vi "Instrument_Setting.vi"(8 "错误输入（无错误）":errorcluster, 9 "id":string[](array[string]), 10 "Get_USB_Resouce":string[](array[string]), 11 "Address Cluster":T2={"SPU"=refnum, "MPM"=[], "Port_Count"=0.0, "MPM_Count"=0.0, "SPU_Resource"=[], "USB_Resource"=[], "MPM_Communicater"="", "MPM_Count"=0.0, "MPM_Address"=[], "MPM_Portnumber"=[], "SPU_DeviveID"="", "MPM_communcation_method"=[], "TSL_sweepstartwave"=0.0, "TSL_sweepstopwave"=0.0, "TSL_Address"="", "TSL_Communicater"="", "TSL"=refnum, "tsl_communcation_method"=3, "TSL_Portnumber"=0.0, "PCU"=refnum, "PCU_Communicater"="", "PCU_Address"="", "PCU_Portnumber"=0.0, "PCU_useing_internal_DAQ"=FALSE, "PCU_communcation_method"=0} {"PCU_communcation_method" items=["GPIB", "C232C", "TCPIP", "USB"]; "tsl_communcation_method" items=["GPIB", "C232C", "TCPIP", "USB"]; "MPM_communcation_method" items=["GPIB", "C232C", "TCPIP", "USB"]}) -> (0 "错误输出":errorcluster, 3 "Address Cluster out":T2={"SPU"=refnum, "MPM"=[], "Port_Count"=0.0, "MPM_Count"=0.0, "SPU_Resource"=[], "USB_Resource"=[], "MPM_Communicater"="", "MPM_Count"=0.0, "MPM_Address"=[], "MPM_Portnumber"=[], "SPU_DeviveID"="", "MPM_communcation_method"=[], "TSL_sweepstartwave"=0.0, "TSL_sweepstopwave"=0.0, "TSL_Address"="", "TSL_Communicater"="", "TSL"=refnum, "tsl_communcation_method"=3, "TSL_Portnumber"=0.0, "PCU"=refnum, "PCU_Communicater"="", "PCU_Address"="", "PCU_Portnumber"=0.0, "PCU_useing_internal_DAQ"=FALSE, "PCU_communcation_method"=0} {"PCU_communcation_method" items=["GPIB", "C232C", "TCPIP", "USB"]; "tsl_communcation_method" items=["GPIB", "C232C", "TCPIP", "USB"]; "MPM_communcation_method" items=["GPIB", "C232C", "TCPIP", "USB"]})   [LabVIEW 2017]
doc: "Setting Form"
uses:
  CTL/Address Cluster.ctl
  D:/test/PDLSTS/LV_PDL_Sample/DLL/InstrumentDLL.dll
  DLL/InstrumentDLL.dll
panel:
  in  "txtpcu_ipadd":string caption="IP Address"
  in  "txtpcu_lanport":i32 caption="LAN Port"
  in  "txtpcu_gpibadd":i32=1 caption="GPIB Address"
  in  "cmbpcu_usbresource":u16(ring) caption="Usb resouce"
  in  "Communication_PCU":T1(radio) caption="Communication"
  in  "Product_PCU":enum32{"rdopcu100", "rdopcu110"}(radio) caption="Product"
  out "Boolean":bool=TRUE
  in  "Port_Count":i32
  in  "btnconnect":bool
  in  "cmbSPU_dev":u16(ring) caption="SPU" items=["Dev8"]
  in  "IP Address_MPM 2":string caption="IP Address"
  in  "LAN Port_MPM 2":dbl caption="LAN Port"
  in  "GPIB Address_MPM 2":i32 caption="GPIB Address"
  in  "chkmulti_dev":bool
  in  "IP Address_MPM":string caption="IP Address"
  in  "LAN Port_MPM":dbl caption="LAN Port"
  in  "GPIB Address_MPM":i32=14 caption="GPIB Address"
  in  "Communication_MPM":enum32{"rdiGPIB_MPM", "rdiLAN_MPM"}(radio) caption="Communication"
  in  "IP Address_TSL1":string caption="IP Address"
  in  "LAN Port_TSL1":i32 caption="LAN Port"
  in  "GPIB Address_TSL1":i32=1 caption="GPIB Address"
  in  "Usb resouce_TSL1":u16(ring) caption="Usb resouce"
  in  "Communication_TSL1":T3(radio) caption="Communication"
  in  "Product_TSL1":enum32{"rdo550_TSL1", "rdo570_TSL1"}(radio) caption="Product"
  # "TSL"
  # "MPM"
  # "Device1"
  # "Device2"
  # "PCU"
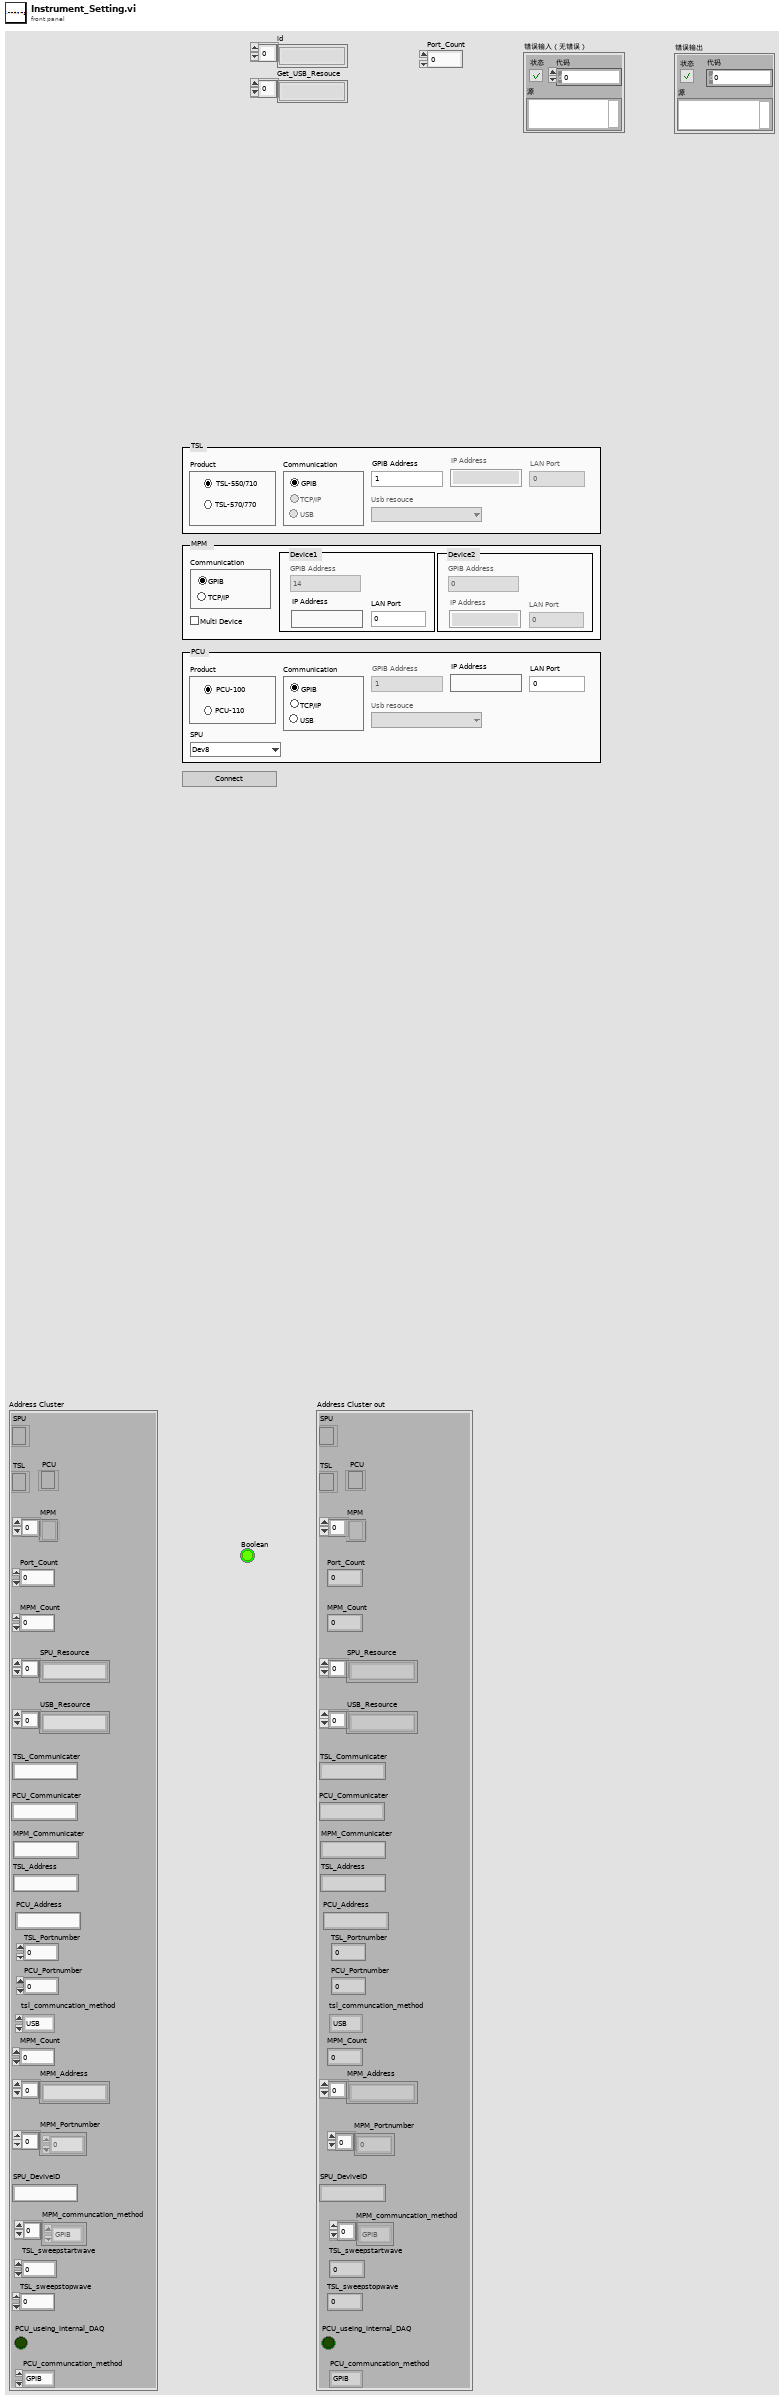
[diagram p1: front panel]
types:
  T1 = enum32{"rdopcu_gpib", "rdopcu_lan", "rdopcu_usb"}
  T2 = typedef "Address Cluster.ctl" = cluster{"SPU":refnum<k24>, "MPM":refnum<k24>[], "Port_Count":dbl, "MPM_Count":dbl, "SPU_Resource":string[], "USB_Resource":string[], "MPM_Communicater":string, "MPM_Count":dbl, "MPM_Address":string[], "MPM_Portnumber":dbl[], "SPU_DeviveID":string, "MPM_communcation_method":i32[], "TSL_sweepstartwave":dbl, "TSL_sweepstopwave":dbl, "TSL_Address":string, "TSL_Communicater":string, "TSL":refnum<k24>, "tsl_communcation_method":i32, "TSL_Portnumber":dbl, "PCU":refnum<k24>, "PCU_Communicater":string, "PCU_Address":string, "PCU_Portnumber":dbl, "PCU_useing_internal_DAQ":bool, "PCU_communcation_method":i32}
  T3 = enum32{"rdiGPIB_TSL1", "rdiLAN_TSL1", "rdiUSB_TSL1"}
  T4 = enum8{"Enabled", "Disabled", "Disabled and Grayed Out"}
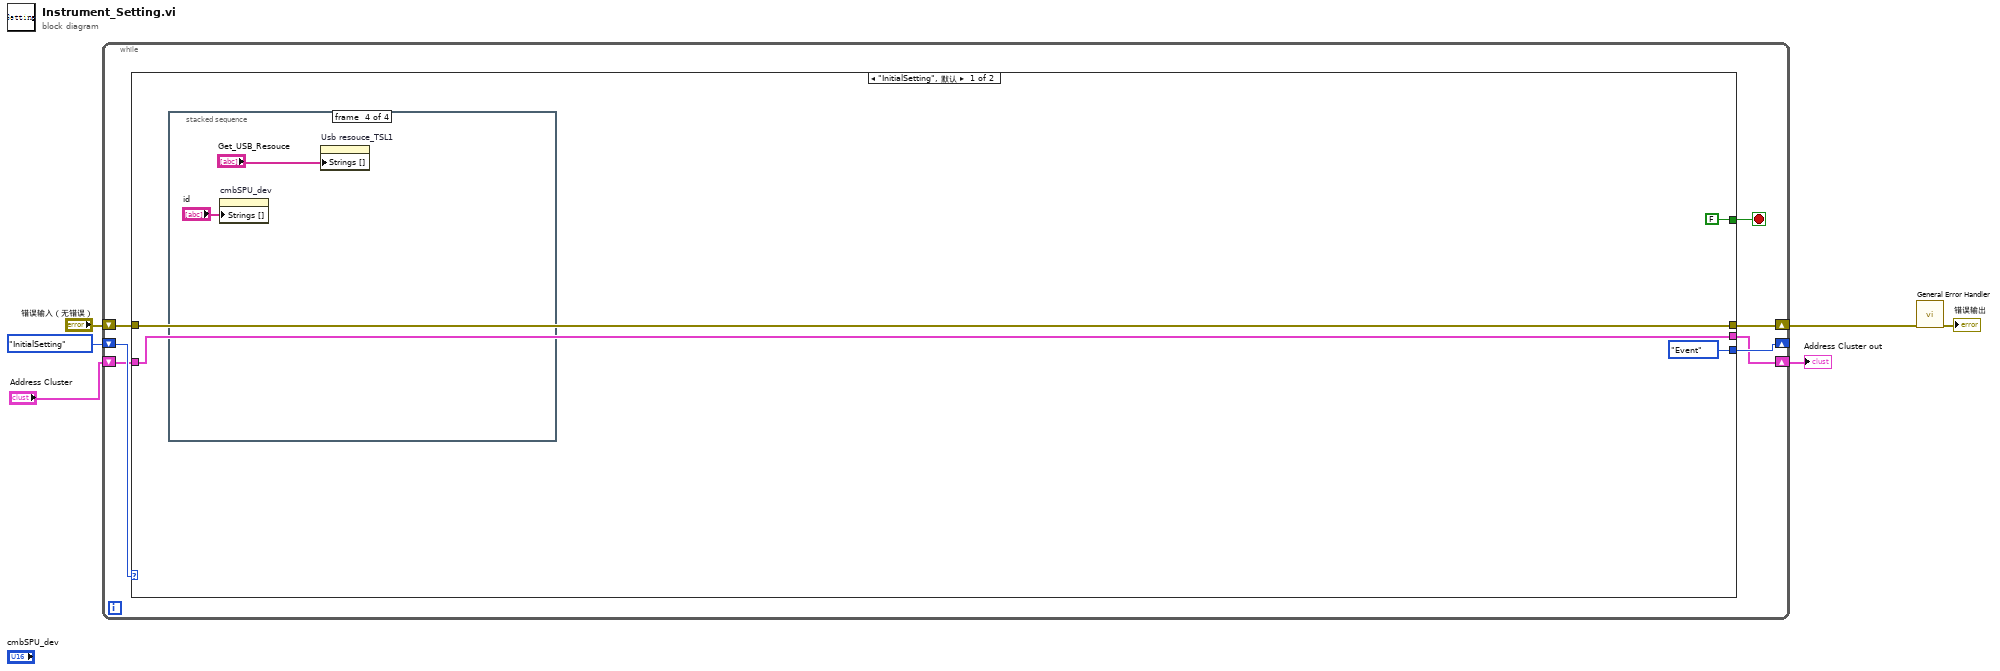
[diagram p0: block diagram]
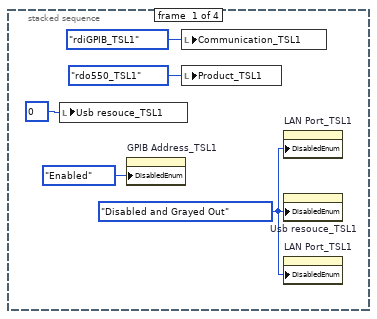
[diagram p2: hidden frame]
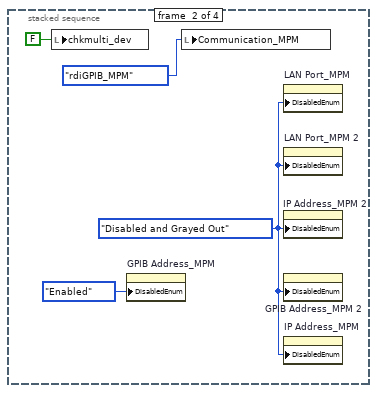
[diagram p3: hidden frame]
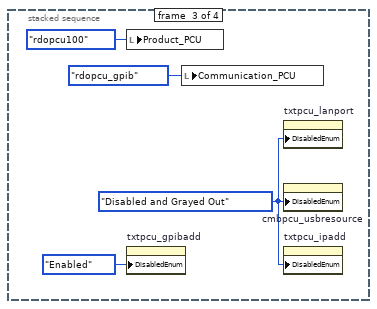
[diagram p4: hidden frame]
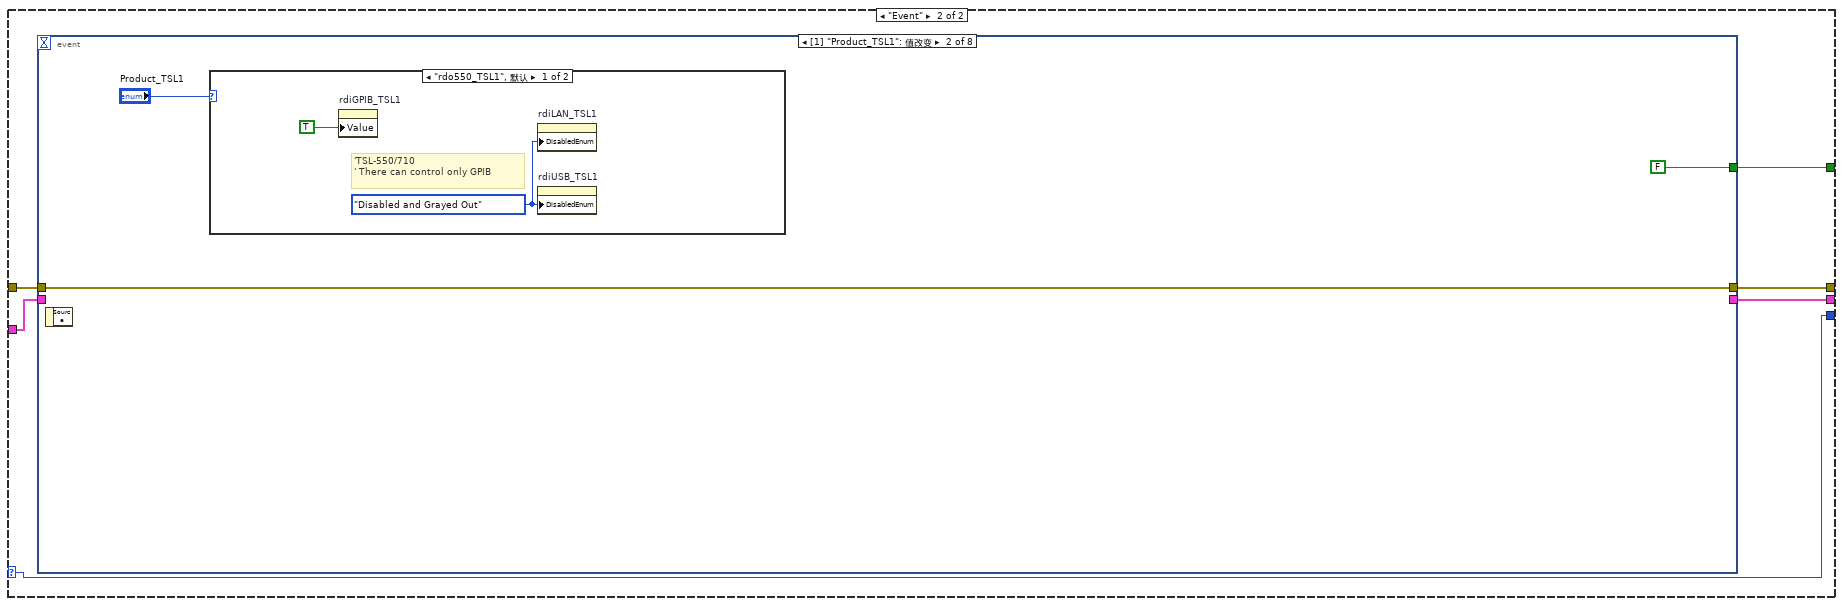
[diagram p5: hidden frame]
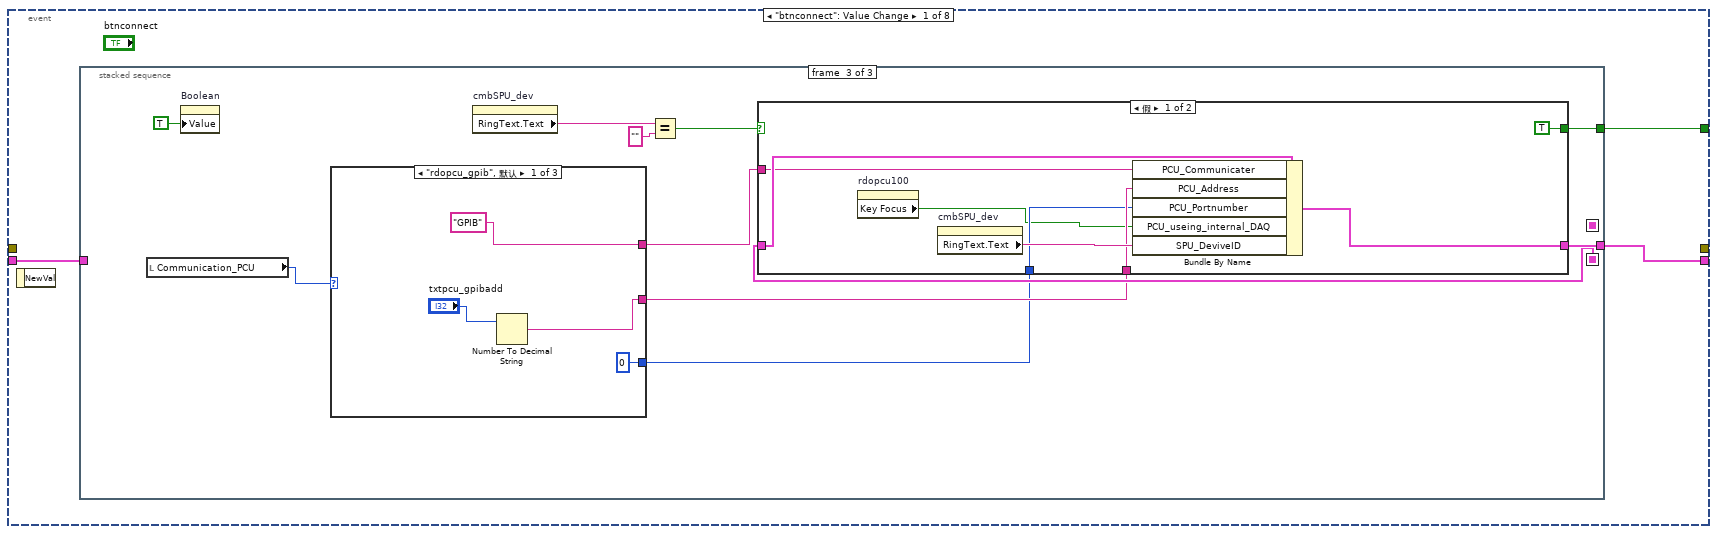
[diagram p6: hidden frame]
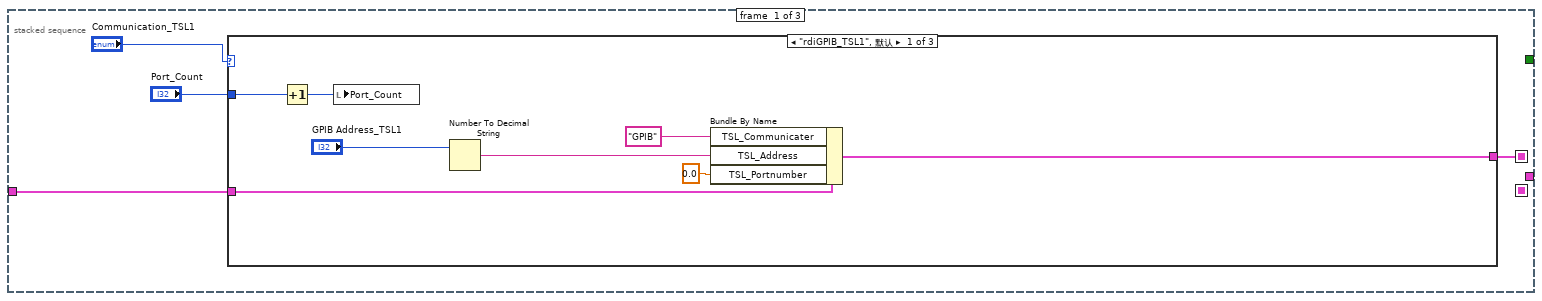
[diagram p7: hidden frame]
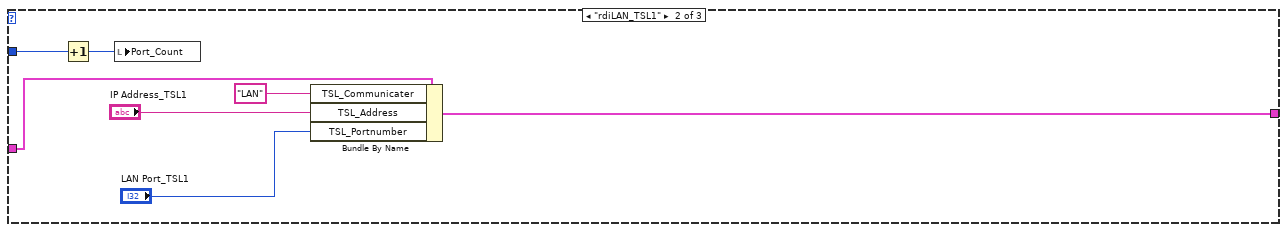
[diagram p8: hidden frame]
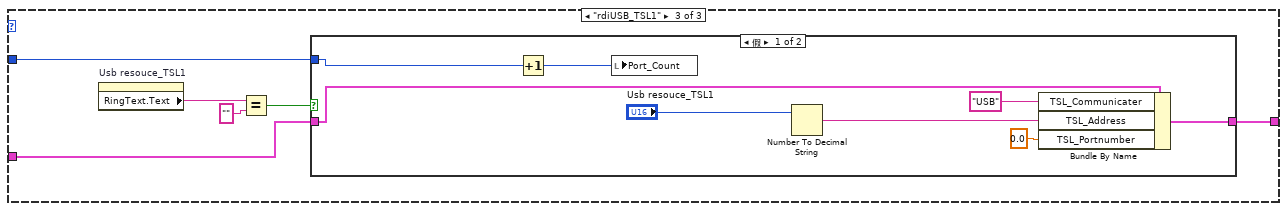
[diagram p9: hidden frame]
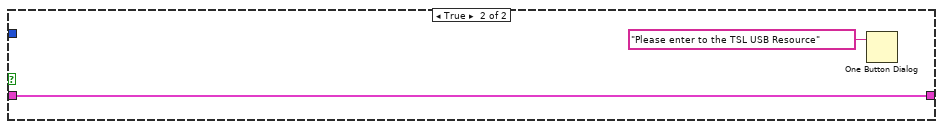
[diagram p10: hidden frame]
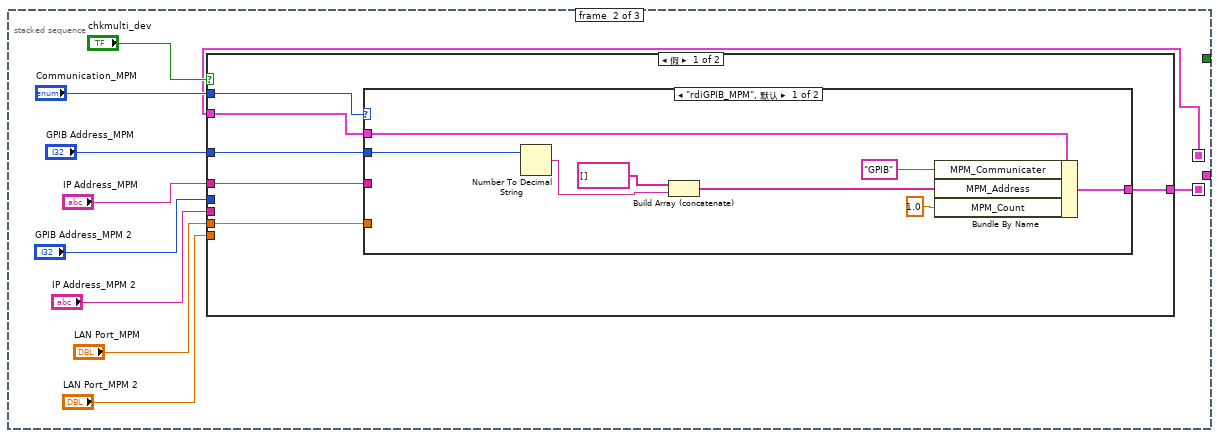
[diagram p11: hidden frame]
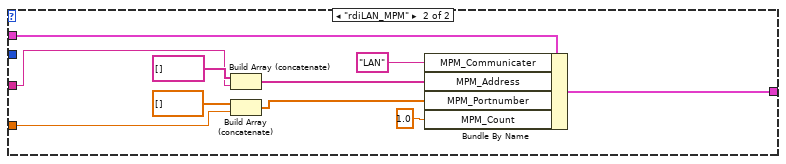
[diagram p12: hidden frame]
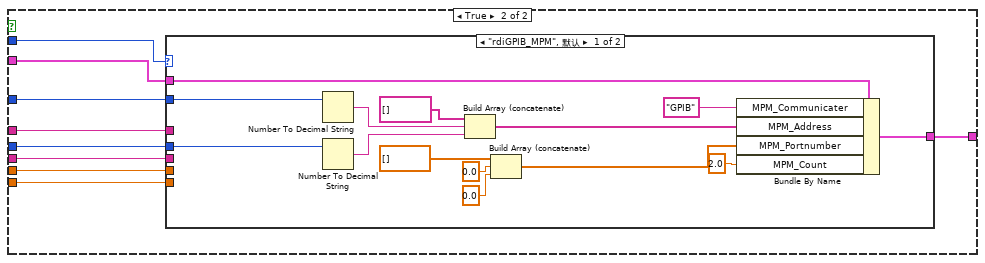
[diagram p13: hidden frame]
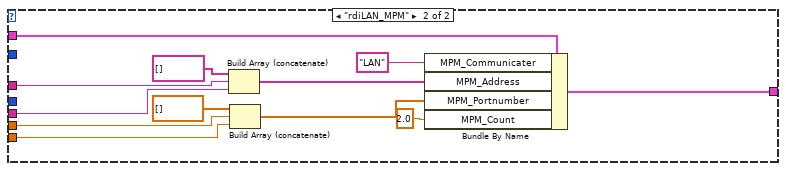
[diagram p14: hidden frame]
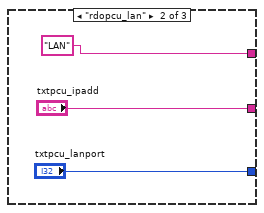
[diagram p15: hidden frame]
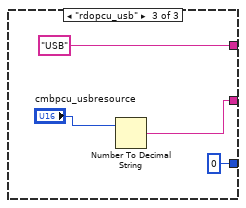
[diagram p16: hidden frame]
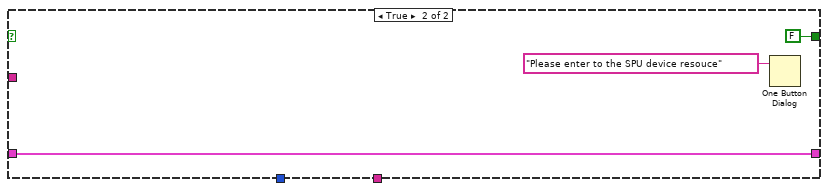
[diagram p17: hidden frame]
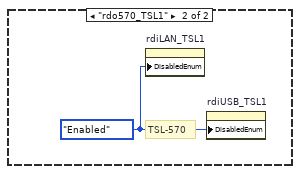
[diagram p18: hidden frame]
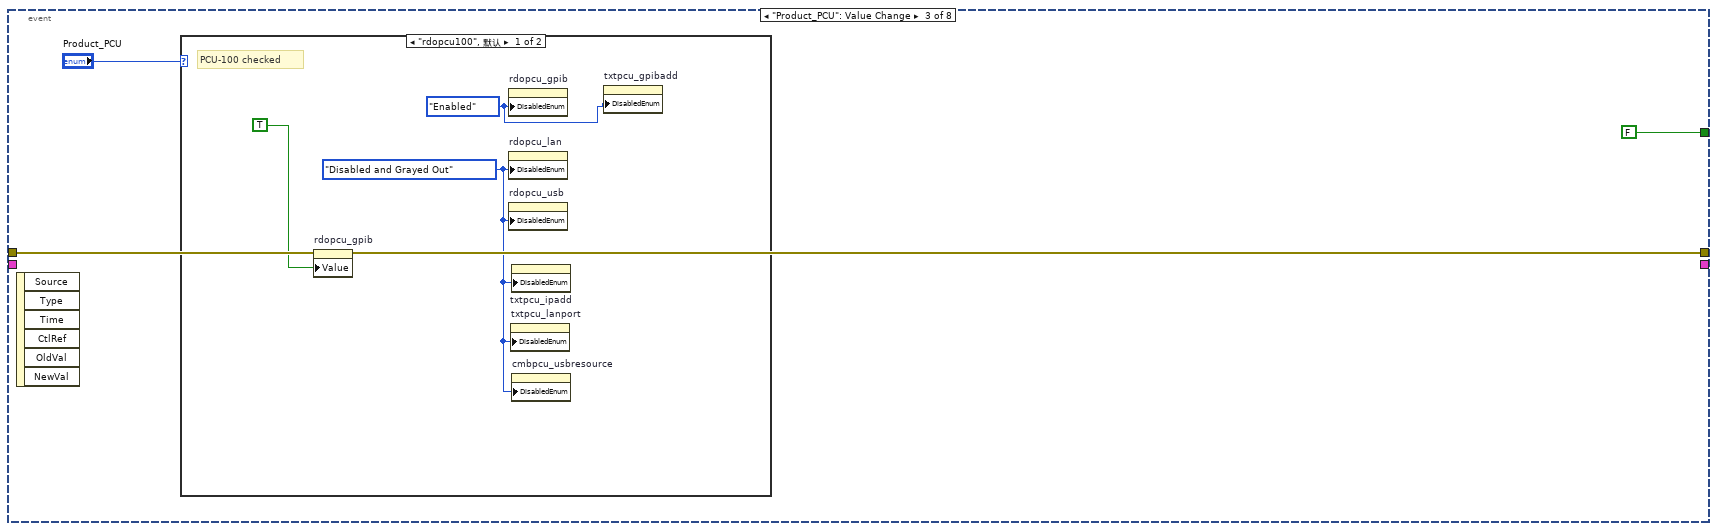
[diagram p19: hidden frame]
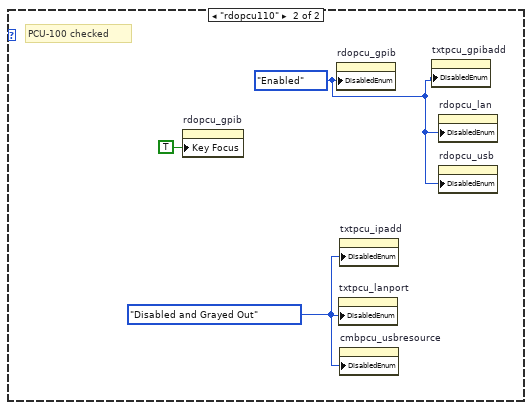
[diagram p20: hidden frame]
diagram:
  n1 = while {
    shift-right: [w12] -> w4
    shift-left: "错误输入（无错误）" -> [w13]
    shift-right: [w10] -> _
    shift-left: enum16{"InitialSetting", "Event", "Set", "Exit"}."InitialSetting" -> [w11]
    shift-right: [w8] -> w1
    shift-left: "Address Cluster" -> [w9]
    stop <- w7 stop-if-true
    n2 = case shown="\"InitialSetting\", 默认" w11 {
      selector: w11 -> [_ w34]
      tunnel: w13 -> [w14 w38]
      tunnel: [w14 w37] -> w12
      tunnel: [FALSE ("status") w33] -> w7
      tunnel: [enum16{"InitialSetting", "Event", "Set", "Exit"}."Event" w34] -> w10
      tunnel: w9 -> [w15 w36]
      tunnel: [w15 w35] -> w8
      frame "InitialSetting", Default {
        n3 = stacked-sequence {
          frame #0 {
            w19 = T4."Disabled and Grayed Out" ("禁用")
            w20 = u16 0 items=[""] ("Usb resouce_TSL1")
            n4 = local write "Usb resouce_TSL1"(w20) -> ()
            n5 = property on="GPIB Address_TSL1" class="DigNum (严格)"("DisabledEnum"=T4."Enabled" ("禁用")) -> ()  [unwired: 2 in, 2 out]
            n6 = local write "Communication_TSL1"(T3."rdiGPIB_TSL1" ("Communication_TSL1")) -> ()
            n7 = local write "Product_TSL1"(enum32{"rdo550_TSL1", "rdo570_TSL1"}."rdo550_TSL1" ("Product_TSL1")) -> ()
            n8 = property on="LAN Port_TSL1" class="DigNum (严格)"("DisabledEnum"=w19) -> ()  [unwired: 2 in, 2 out]
            n9 = property on="Usb resouce_TSL1" class="Ring (严格)"("DisabledEnum"=w19) -> ()  [unwired: 2 in, 2 out]
            n10 = property on="LAN Port_TSL1" class="DigNum (严格)"("DisabledEnum"=w19) -> ()  [unwired: 2 in, 2 out]
          }
          frame #1 {
            w23 = T4."Disabled and Grayed Out" ("禁用")
            n11 = local write "chkmulti_dev"(FALSE ("chkmulti_dev")) -> ()
            n12 = property on="GPIB Address_MPM" class="DigNum (严格)"("DisabledEnum"=T4."Enabled" ("禁用")) -> ()  [unwired: 2 in, 2 out]
            n13 = local write "Communication_MPM"(enum32{"rdiGPIB_MPM", "rdiLAN_MPM"}."rdiGPIB_MPM" ("Communication_MPM")) -> ()
            n14 = property on="LAN Port_MPM" class="DigNum (严格)"("DisabledEnum"=w23) -> ()  [unwired: 2 in, 2 out]
            n15 = property on="LAN Port_MPM 2" class="DigNum (严格)"("DisabledEnum"=w23) -> ()  [unwired: 2 in, 2 out]
            n16 = property on="IP Address_MPM 2" class="Str"("DisabledEnum"=w23) -> ()  [unwired: 2 in, 2 out]
            n17 = property on="GPIB Address_MPM 2" class="DigNum (严格)"("DisabledEnum"=w23) -> ()  [unwired: 2 in, 2 out]
            n18 = property on="IP Address_MPM" class="Str"("DisabledEnum"=w23) -> ()  [unwired: 2 in, 2 out]
          }
          frame #2 {
            w27 = T4."Disabled and Grayed Out" ("禁用")
            n19 = local write "Product_PCU"(enum32{"rdopcu100", "rdopcu110"}."rdopcu100" ("Product_PCU")) -> ()
            n20 = property on="txtpcu_gpibadd" class="DigNum (严格)"("DisabledEnum"=T4."Enabled" ("禁用")) -> ()  [unwired: 2 in, 2 out]
            n21 = local write "Communication_PCU"(T1."rdopcu_gpib" ("Communication_PCU")) -> ()
            n22 = property on="txtpcu_lanport" class="DigNum (严格)"("DisabledEnum"=w27) -> ()  [unwired: 2 in, 2 out]
            n23 = property on="cmbpcu_usbresource" class="Ring (严格)"("DisabledEnum"=w27) -> ()  [unwired: 2 in, 2 out]
            n24 = property on="txtpcu_ipadd" class="Str"("DisabledEnum"=w27) -> ()  [unwired: 2 in, 2 out]
          }
          frame #3 {
            n25 = property on="cmbSPU_dev" class="Ring (严格)"("Strings []"="id") -> ()  [unwired: 2 in, 2 out]
            n26 = property on="Usb resouce_TSL1" class="Ring (严格)"("Strings []"="Get_USB_Resouce") -> ()  [unwired: 2 in, 2 out]
          }
        }
      }
      frame "Event" {
        n27 = event shown="[1] \"Product_TSL1\": 值改变" {
          selector: _ -> [_ _ _ _ _ _ _ _]
          dyn-events: _ -> [_ _ _ _ _ _ _ _]
          timeout: _ -> [_ _ _ _ _ _ _ _]
          tunnel: w38 -> [_ w179 w186 w194 _ w210 w219 _]
          tunnel: [_ w179 w186 w194 _ w210 w219 _] -> w37
          tunnel: w36 -> [w41 _ _ _ _ _ _ w234]
          tunnel: [w40 _ _ _ _ _ _ w234] -> w35
          tunnel: [w39 FALSE ("y") FALSE ("y") FALSE ("y") _ FALSE ("y") FALSE ("y") TRUE ("y")] -> w33
          event "btnconnect": Value Change {
            n28 = event-data() -> ()  [unwired: 1 in, 1 out]
            n29 = stacked-sequence {
              seq-local: [w44 _ _] -> [_ w77 _]
              seq-local: [_ w78 _] -> [_ _ w151]
              tunnel: w41 -> [w45 _ _]
              tunnel: [_ _ w153] -> w40
              tunnel: [_ _ w152] -> w39
              frame #0 {
                n30 = case shown="\"rdiGPIB_TSL1\", 默认" "Communication_TSL1" {
                  tunnel: "Port_Count" -> [w49 w58 w63]
                  tunnel: w45 -> [w52 w60 w62]
                  tunnel: [w51 w59 w61] -> w44
                  frame "rdiGPIB_TSL1", Default {
                    n31 = Increment(x=w49) -> (x+1=w50:i32)
                    n32 = local write "Port_Count"(w50) -> ()
                    n33 = Number To Decimal String(number="GPIB Address_TSL1") -> (decimal integer string=w47:string)  [unwired: 1 in]
                    n34 = Bundle By Name(cluster=w52, "TSL_Communicater"="GPIB" ("新元素/子数组"), "TSL_Address"=w47, "TSL_Portnumber"=0.0 ("新元素/子数组")) -> (w51:T2)
                  }
                  frame "rdiLAN_TSL1" {
                    n35 = Increment(x=w58) -> (x+1=w57:i32)
                    n36 = local write "Port_Count"(w57) -> ()
                    n37 = Bundle By Name(cluster=w60, "TSL_Communicater"="LAN" ("新元素/子数组"), "TSL_Address"="IP Address_TSL1", "TSL_Portnumber"="LAN Port_TSL1") -> (w59:T2)
                  }
                  frame "rdiUSB_TSL1" {
                    n38 = property on="Usb resouce_TSL1" class="Ring (严格)"() -> ("RingText.Text"=w66:string)  [unwired: 2 in, 2 out]
                    n39 = Equal?(x=w66, y="") -> (x = y?=w64:bool)
                    n40 = case shown="假" w64 {
                      tunnel: w63 -> [w70 _]
                      tunnel: w62 -> [w73 w75]
                      tunnel: [w72 w75] -> w61
                      frame False {
                        n41 = Increment(x=w70) -> (x+1=w71:i32)
                        n42 = local write "Port_Count"(w71) -> ()
                        n43 = Number To Decimal String(number="Usb resouce_TSL1") -> (decimal integer string=w68:string)  [unwired: 1 in]
                        n44 = Bundle By Name(cluster=w73, "TSL_Communicater"="USB" ("新元素/子数组"), "TSL_Address"=w68, "TSL_Portnumber"=0.0 ("新元素/子数组")) -> (w72:T2)
                      }
                      frame True {
                        n45 = One Button Dialog(message="Please enter to the TSL USB Resource" ("消息")) -> ()  [unwired: 1 in, 1 out]
                      }
                    }
                  }
                }
              }
              frame #1 {
                n46 = case shown="假" "chkmulti_dev" {
                  tunnel: w77 -> [w88 w119]
                  tunnel: "Communication_MPM" -> [w92 w118]
                  tunnel: [w89 w117] -> w78
                  tunnel: "GPIB Address_MPM 2" -> [_ w116]
                  tunnel: "GPIB Address_MPM" -> [w87 w115]
                  tunnel: "LAN Port_MPM 2" -> [_ w114]
                  tunnel: "LAN Port_MPM" -> [w91 w113]
                  tunnel: "IP Address_MPM 2" -> [_ w112]
                  tunnel: "IP Address_MPM" -> [w90 w111]
                  frame False {
                    n47 = case shown="\"rdiGPIB_MPM\", 默认" w92 {
                      tunnel: w91 -> [_ w107]
                      tunnel: w90 -> [_ w104]
                      tunnel: [w97 w102] -> w89
                      tunnel: w88 -> [w98 w101]
                      tunnel: w87 -> [w94 _]
                      frame "rdiGPIB_MPM", Default {
                        n48 = Number To Decimal String(number=w94) -> (decimal integer string=w95:string)  [unwired: 1 in]
                        n49 = Build Array (concatenate)(string[] [] ("MPM_Address"), w95) -> (w93:string[])
                        n50 = Bundle By Name(cluster=w98, "MPM_Communicater"="GPIB", "MPM_Address"=w93, "MPM_Count"=1.0) -> (w97:T2)
                      }
                      frame "rdiLAN_MPM" {
                        n51 = Build Array (concatenate)(string[] [] ("MPM_Address"), w104) -> (w103:string[])
                        n52 = Build Array (concatenate)(dbl[] [] ("MPM_Portnumber"), w107) -> (w106:dbl[])
                        n53 = Bundle By Name(cluster=w101, "MPM_Communicater"="LAN", "MPM_Address"=w103, "MPM_Portnumber"=w106, "MPM_Count"=1.0) -> (w102:T2)
                      }
                    }
                  }
                  frame True {
                    n54 = case shown="\"rdiGPIB_MPM\", 默认" w118 {
                      tunnel: w119 -> [w127 w145]
                      tunnel: [w122 w134] -> w117
                      tunnel: w116 -> [w121 _]
                      tunnel: w115 -> [w120 _]
                      tunnel: w114 -> [_ w138]
                      tunnel: w113 -> [_ w137]
                      tunnel: w112 -> [_ w136]
                      tunnel: w111 -> [_ w135]
                      frame "rdiGPIB_MPM", Default {
                        n55 = Number To Decimal String(number=w120) -> (decimal integer string=w130:string)  [unwired: 1 in]
                        n56 = Number To Decimal String(number=w121) -> (decimal integer string=w129:string)  [unwired: 1 in]
                        n57 = Build Array (concatenate)(string[] [] ("MPM_Address"), w130, w129) -> (w128:string[])
                        n58 = Build Array (concatenate)(dbl[] [] ("MPM_Portnumber"), 0.0 ("新元素/子数组"), 0.0 ("新元素/子数组")) -> (w123:dbl[])
                        n59 = Bundle By Name(cluster=w127, "MPM_Communicater"="GPIB", "MPM_Address"=w128, "MPM_Portnumber"=w123, "MPM_Count"=2.0) -> (w122:T2)
                      }
                      frame "rdiLAN_MPM" {
                        n60 = Build Array (concatenate)(string[] [] ("MPM_Address"), w135, w136) -> (w141:string[])
                        n61 = Build Array (concatenate)(dbl[] [] ("MPM_Portnumber"), w137, w138) -> (w139:dbl[])
                        n62 = Bundle By Name(cluster=w145, "MPM_Communicater"="LAN", "MPM_Address"=w141, "MPM_Portnumber"=w139, "MPM_Count"=2.0) -> (w134:T2)
                      }
                    }
                  }
                }
              }
              frame #2 {
                n63 = local read "Communication_PCU"() -> (w149:T1)
                n64 = property on="Boolean" class="Bool (严格)"("Value"=TRUE ("Boolean")) -> ()  [unwired: 2 in, 2 out]
                n65 = case shown="\"rdopcu_gpib\", 默认" w149 {
                  tunnel: ["GPIB" "LAN" "USB"] -> w148
                  tunnel: [w158 "txtpcu_ipadd" w165] -> w147
                  tunnel: [0 ("txtpcu_lanport") "txtpcu_lanport" 0 ("txtpcu_lanport")] -> w146
                  frame "rdopcu_gpib", Default {
                    n66 = Number To Decimal String(number="txtpcu_gpibadd") -> (decimal integer string=w158:string)  [unwired: 1 in]
                  }
                  frame "rdopcu_lan" {
                  }
                  frame "rdopcu_usb" {
                    n67 = Number To Decimal String(number="cmbpcu_usbresource") -> (decimal integer string=w165:string)  [unwired: 1 in]
                  }
                }
                n68 = property on="cmbSPU_dev" class="Ring (严格)"() -> ("RingText.Text"=w155:string)  [unwired: 2 in, 2 out]
                n69 = Equal?(x=w155, y="") -> (x = y?=w156:bool)
                n70 = case shown="假" w156 {
                  tunnel: w151 -> [w175 w177]
                  tunnel: [w174 w177] -> w153
                  tunnel: [TRUE ("y") FALSE ("y")] -> w152
                  tunnel: w148 -> [w171 _]
                  tunnel: w147 -> [w170 _]
                  tunnel: w146 -> [w169 _]
                  frame False {
                    n71 = property on="rdopcu100" class="Bool (严格)"() -> ("Key Focus"=w168:bool)  [unwired: 2 in, 2 out]
                    n72 = property on="cmbSPU_dev" class="Ring (严格)"() -> ("RingText.Text"=w173:string)  [unwired: 2 in, 2 out]
                    n73 = Bundle By Name(cluster=w175, "PCU_Communicater"=w171, "PCU_Address"=w170, "PCU_Portnumber"=w169, "PCU_useing_internal_DAQ"=w168, "SPU_DeviveID"=w173) -> (w174:T2)
                  }
                  frame True {
                    n74 = One Button Dialog(message="Please enter to the SPU device resouce" ("消息")) -> ()  [unwired: 1 in, 1 out]
                  }
                }
              }
            }
          }
          event "Product_TSL1": Value Change {
            n75 = event-data() -> ()  [unwired: 1 in, 1 out]
            n76 = case shown="\"rdo550_TSL1\", 默认" "Product_TSL1" {
              frame "rdo550_TSL1", Default {
                w183 = T4."Disabled and Grayed Out" ("禁用")
                # "'TSL-550/710\n' There can control only GPIB"
                n77 = property on="rdiGPIB_TSL1" class="Bool (严格)"("Value"=TRUE ("键选中")) -> ()  [unwired: 2 in, 2 out]
                n78 = property on="rdiLAN_TSL1" class="Bool (严格)"("DisabledEnum"=w183) -> ()  [unwired: 2 in, 2 out]
                n79 = property on="rdiUSB_TSL1" class="Bool (严格)"("DisabledEnum"=w183) -> ()  [unwired: 2 in, 2 out]
              }
              frame "rdo570_TSL1" {
                w184 = T4."Enabled" ("禁用")
                # "TSL-570"
                n80 = property on="rdiLAN_TSL1" class="Bool (严格)"("DisabledEnum"=w184) -> ()  [unwired: 2 in, 2 out]
                n81 = property on="rdiUSB_TSL1" class="Bool (严格)"("DisabledEnum"=w184) -> ()  [unwired: 2 in, 2 out]
              }
            }
          }
          event "Product_PCU": Value Change {
            n82 = event-data() -> ()  [unwired: 1 in, 6 out]
            n83 = case shown="\"rdopcu100\", 默认" "Product_PCU" {
              frame "rdopcu100", Default {
                w189 = T4."Enabled" ("禁用")
                w190 = T4."Disabled and Grayed Out" ("禁用")
                # "PCU-100 checked"
                n84 = property on="rdopcu_gpib" class="Bool (严格)"("Value"=TRUE ("键选中")) -> ()  [unwired: 2 in, 2 out]
                n85 = property on="rdopcu_gpib" class="Bool (严格)"("DisabledEnum"=w189) -> ()  [unwired: 2 in, 2 out]
                n86 = property on="rdopcu_lan" class="Bool (严格)"("DisabledEnum"=w190) -> ()  [unwired: 2 in, 2 out]
                n87 = property on="rdopcu_usb" class="Bool (严格)"("DisabledEnum"=w190) -> ()  [unwired: 2 in, 2 out]
                n88 = property on="txtpcu_lanport" class="DigNum (严格)"("DisabledEnum"=w190) -> ()  [unwired: 2 in, 2 out]
                n89 = property on="txtpcu_ipadd" class="Str"("DisabledEnum"=w190) -> ()  [unwired: 2 in, 2 out]
                n90 = property on="cmbpcu_usbresource" class="Ring (严格)"("DisabledEnum"=w190) -> ()  [unwired: 2 in, 2 out]
                n91 = property on="txtpcu_gpibadd" class="DigNum (严格)"("DisabledEnum"=w189) -> ()  [unwired: 2 in, 2 out]
              }
              frame "rdopcu110" {
                w192 = T4."Enabled" ("禁用")
                w193 = T4."Disabled and Grayed Out" ("禁用")
                # "PCU-100 checked"
                n92 = property on="rdopcu_gpib" class="Bool (严格)"("Key Focus"=TRUE ("键选中")) -> ()  [unwired: 2 in, 2 out]
                n93 = property on="rdopcu_gpib" class="Bool (严格)"("DisabledEnum"=w192) -> ()  [unwired: 2 in, 2 out]
                n94 = property on="txtpcu_lanport" class="DigNum (严格)"("DisabledEnum"=w193) -> ()  [unwired: 2 in, 2 out]
                n95 = property on="txtpcu_ipadd" class="Str"("DisabledEnum"=w193) -> ()  [unwired: 2 in, 2 out]
                n96 = property on="cmbpcu_usbresource" class="Ring (严格)"("DisabledEnum"=w193) -> ()  [unwired: 2 in, 2 out]
                n97 = property on="txtpcu_gpibadd" class="DigNum (严格)"("DisabledEnum"=w192) -> ()  [unwired: 2 in, 2 out]
                n98 = property on="rdopcu_lan" class="Bool (严格)"("DisabledEnum"=w192) -> ()  [unwired: 2 in, 2 out]
                n99 = property on="rdopcu_usb" class="Bool (严格)"("DisabledEnum"=w192) -> ()  [unwired: 2 in, 2 out]
              }
            }
          }
          event "Communication_TSL1": Value Change {
            n100 = event-data() -> ()  [unwired: 1 in, 1 out]
            n101 = local read "Communication_TSL1"() -> (w196:T3)
            n102 = case shown="\"rdiGPIB_TSL1\", 默认" w196 {
              frame "rdiLAN_TSL1" {
                w197 = T4."Enabled" ("禁用")
                w198 = T4."Disabled and Grayed Out" ("禁用")
                # "TSL Control TCP/IP"
                n103 = property on="IP Address_TSL1" class="Str"("DisabledEnum"=w197) -> ()  [unwired: 2 in, 2 out]
                n104 = property on="LAN Port_TSL1" class="DigNum (严格)"("DisabledEnum"=w197) -> ()  [unwired: 2 in, 2 out]
                n105 = property on="Usb resouce_TSL1" class="Ring (严格)"("DisabledEnum"=w198) -> ()  [unwired: 2 in, 2 out]
                n106 = property on="GPIB Address_TSL1" class="DigNum (严格)"("DisabledEnum"=w198) -> ()  [unwired: 2 in, 2 out]
              }
              frame "rdiGPIB_TSL1", Default {
                w199 = T4."Disabled and Grayed Out" ("禁用")
                # "TSL Control GPIB"
                n107 = property on="GPIB Address_TSL1" class="DigNum (严格)"("DisabledEnum"=T4."Enabled" ("禁用")) -> ()  [unwired: 2 in, 2 out]
                n108 = property on="Usb resouce_TSL1" class="Ring (严格)"("DisabledEnum"=w199) -> ()  [unwired: 2 in, 2 out]
                n109 = property on="LAN Port_TSL1" class="DigNum (严格)"("DisabledEnum"=w199) -> ()  [unwired: 2 in, 2 out]
                n110 = property on="IP Address_TSL1" class="Str"("DisabledEnum"=w199) -> ()  [unwired: 2 in, 2 out]
              }
              frame "rdiUSB_TSL1" {
                w201 = T4."Disabled and Grayed Out" ("禁用")
                # "TSL Control USB"
                n111 = property on="Usb resouce_TSL1" class="Ring (严格)"("DisabledEnum"=T4."Enabled" ("禁用")) -> ()  [unwired: 2 in, 2 out]
                n112 = property on="GPIB Address_TSL1" class="DigNum (严格)"("DisabledEnum"=w201) -> ()  [unwired: 2 in, 2 out]
                n113 = property on="LAN Port_TSL1" class="DigNum (严格)"("DisabledEnum"=w201) -> ()  [unwired: 2 in, 2 out]
                n114 = property on="IP Address_TSL1" class="Str"("DisabledEnum"=w201) -> ()  [unwired: 2 in, 2 out]
              }
            }
          }
          event "Communication_PCU": Value Change {
            n115 = event-data() -> ()  [unwired: 1 in, 6 out]
            n116 = case shown="\"rdopcu_gpib\", 默认" "Communication_PCU" {
              frame "rdopcu_gpib", Default {
                w204 = T4."Disabled and Grayed Out" ("禁用")
                # "PCU Communcatior GPIB Checked"
                n117 = property on="txtpcu_ipadd" class="Str"("DisabledEnum"=w204) -> ()  [unwired: 2 in, 2 out]
                n118 = property on="txtpcu_gpibadd" class="DigNum (严格)"("DisabledEnum"=T4."Enabled" ("禁用")) -> ()  [unwired: 2 in, 2 out]
                n119 = property on="txtpcu_lanport" class="DigNum (严格)"("DisabledEnum"=w204) -> ()  [unwired: 2 in, 2 out]
                n120 = property on="cmbpcu_usbresource" class="Ring (严格)"("DisabledEnum"=w204) -> ()  [unwired: 2 in, 2 out]
              }
              frame "rdopcu_usb" {
                w207 = T4."Disabled and Grayed Out" ("禁用")
                # "PCU Communicator USB checked"
                n121 = property on="txtpcu_ipadd" class="Str"("DisabledEnum"=w207) -> ()  [unwired: 2 in, 2 out]
                n122 = property on="txtpcu_lanport" class="DigNum (严格)"("DisabledEnum"=w207) -> ()  [unwired: 2 in, 2 out]
                n123 = property on="txtpcu_gpibadd" class="DigNum (严格)"("DisabledEnum"=w207) -> ()  [unwired: 2 in, 2 out]
                n124 = property on="cmbpcu_usbresource" class="Ring (严格)"("DisabledEnum"=T4."Enabled" ("禁用")) -> ()  [unwired: 2 in, 2 out]
              }
              frame "rdopcu_lan" {
                w209 = T4."Disabled and Grayed Out" ("禁用")
                w208 = T4."Enabled" ("禁用")
                # "PCU communcatior TCP/IP Checked"
                n125 = property on="cmbpcu_usbresource" class="Ring (严格)"("DisabledEnum"=w209) -> ()  [unwired: 2 in, 2 out]
                n126 = property on="txtpcu_gpibadd" class="DigNum (严格)"("DisabledEnum"=w209) -> ()  [unwired: 2 in, 2 out]
                n127 = property on="txtpcu_ipadd" class="Str"("DisabledEnum"=w208) -> ()  [unwired: 2 in, 2 out]
                n128 = property on="txtpcu_lanport" class="DigNum (严格)"("DisabledEnum"=w208) -> ()  [unwired: 2 in, 2 out]
              }
            }
          }
          event "chkmulti_dev": Value Change {
            n129 = event-data() -> ()  [unwired: 1 in, 1 out]
            n130 = local read "chkmulti_dev"() -> (w212:bool)
            n131 = case shown="真" w212 {
              frame False {
                w213 = T4."Disabled and Grayed Out" ("禁用")
                n132 = property on="LAN Port_MPM 2" class="DigNum (严格)"("DisabledEnum"=w213) -> ()  [unwired: 2 in, 2 out]
                n133 = property on="IP Address_MPM 2" class="Str"("DisabledEnum"=w213) -> ()  [unwired: 2 in, 2 out]
                n134 = property on="GPIB Address_MPM 2" class="DigNum (严格)"("DisabledEnum"=w213) -> ()  [unwired: 2 in, 2 out]
              }
              frame True {
                n135 = local read "Communication_MPM"() -> (w214:enum32{"rdiGPIB_MPM", "rdiLAN_MPM"})
                n136 = case shown="\"rdiGPIB_MPM\", 默认" w214 {
                  frame "rdiLAN_MPM" {
                    w215 = T4."Enabled" ("禁用")
                    n137 = property on="LAN Port_MPM 2" class="DigNum (严格)"("DisabledEnum"=w215) -> ()  [unwired: 2 in, 2 out]
                    n138 = property on="IP Address_MPM 2" class="Str"("DisabledEnum"=w215) -> ()  [unwired: 2 in, 2 out]
                    n139 = property on="GPIB Address_MPM 2" class="DigNum (严格)"("DisabledEnum"=T4."Disabled and Grayed Out" ("禁用")) -> ()  [unwired: 2 in, 2 out]
                  }
                  frame "rdiGPIB_MPM", Default {
                    w217 = T4."Disabled and Grayed Out" ("禁用")
                    n140 = property on="GPIB Address_MPM 2" class="DigNum (严格)"("DisabledEnum"=T4."Enabled" ("禁用")) -> ()  [unwired: 2 in, 2 out]
                    n141 = property on="IP Address_MPM 2" class="Str"("DisabledEnum"=w217) -> ()  [unwired: 2 in, 2 out]
                    n142 = property on="LAN Port_MPM 2" class="DigNum (严格)"("DisabledEnum"=w217) -> ()  [unwired: 2 in, 2 out]
                  }
                }
              }
            }
          }
          event "Communication_MPM": Value Change {
            n143 = event-data() -> ()  [unwired: 1 in, 1 out]
            n144 = local read "Communication_MPM"() -> (w221:enum32{"rdiGPIB_MPM", "rdiLAN_MPM"})
            n145 = case shown="\"rdiGPIB_MPM\", 默认" w221 {
              frame "rdiLAN_MPM" {
                n146 = local read "chkmulti_dev"() -> (w222:bool)
                n147 = case shown="真" w222 {
                  frame True {
                    w223 = T4."Disabled and Grayed Out" ("禁用")
                    w224 = T4."Enabled" ("禁用")
                    n148 = property on="IP Address_MPM" class="Str"("DisabledEnum"=w224) -> ()  [unwired: 2 in, 2 out]
                    n149 = property on="LAN Port_MPM" class="DigNum (严格)"("DisabledEnum"=w224) -> ()  [unwired: 2 in, 2 out]
                    n150 = property on="LAN Port_MPM 2" class="DigNum (严格)"("DisabledEnum"=w224) -> ()  [unwired: 2 in, 2 out]
                    n151 = property on="IP Address_MPM 2" class="Str"("DisabledEnum"=w224) -> ()  [unwired: 2 in, 2 out]
                    n152 = property on="GPIB Address_MPM 2" class="DigNum (严格)"("DisabledEnum"=w223) -> ()  [unwired: 2 in, 2 out]
                    n153 = property on="GPIB Address_MPM" class="DigNum (严格)"("DisabledEnum"=w223) -> ()  [unwired: 2 in, 2 out]
                  }
                  frame False {
                    w225 = T4."Disabled and Grayed Out" ("禁用")
                    w226 = T4."Disabled and Grayed Out" ("禁用")
                    w227 = T4."Enabled" ("禁用")
                    n154 = property on="IP Address_MPM" class="Str"("DisabledEnum"=w227) -> ()  [unwired: 2 in, 2 out]
                    n155 = property on="LAN Port_MPM" class="DigNum (严格)"("DisabledEnum"=w227) -> ()  [unwired: 2 in, 2 out]
                    n156 = property on="IP Address_MPM 2" class="Str"("DisabledEnum"=w225) -> ()  [unwired: 2 in, 2 out]
                    n157 = property on="LAN Port_MPM 2" class="DigNum (严格)"("DisabledEnum"=w225) -> ()  [unwired: 2 in, 2 out]
                    n158 = property on="GPIB Address_MPM 2" class="DigNum (严格)"("DisabledEnum"=w226) -> ()  [unwired: 2 in, 2 out]
                    n159 = property on="GPIB Address_MPM" class="DigNum (严格)"("DisabledEnum"=w226) -> ()  [unwired: 2 in, 2 out]
                  }
                }
              }
              frame "rdiGPIB_MPM", Default {
                n160 = local read "chkmulti_dev"() -> (w228:bool)
                n161 = case shown="假" w228 {
                  frame True {
                    w229 = T4."Enabled" ("禁用")
                    w230 = T4."Disabled and Grayed Out" ("禁用")
                    n162 = property on="GPIB Address_MPM" class="DigNum (严格)"("DisabledEnum"=w229) -> ()  [unwired: 2 in, 2 out]
                    n163 = property on="GPIB Address_MPM 2" class="DigNum (严格)"("DisabledEnum"=w229) -> ()  [unwired: 2 in, 2 out]
                    n164 = property on="IP Address_MPM" class="Str"("DisabledEnum"=w230) -> ()  [unwired: 2 in, 2 out]
                    n165 = property on="LAN Port_MPM" class="DigNum (严格)"("DisabledEnum"=w230) -> ()  [unwired: 2 in, 2 out]
                    n166 = property on="IP Address_MPM 2" class="Str"("DisabledEnum"=w230) -> ()  [unwired: 2 in, 2 out]
                    n167 = property on="LAN Port_MPM 2" class="DigNum (严格)"("DisabledEnum"=w230) -> ()  [unwired: 2 in, 2 out]
                  }
                  frame False {
                    w231 = T4."Disabled and Grayed Out" ("禁用")
                    n168 = property on="GPIB Address_MPM" class="DigNum (严格)"("DisabledEnum"=T4."Enabled" ("禁用")) -> ()  [unwired: 2 in, 2 out]
                    n169 = property on="GPIB Address_MPM 2" class="DigNum (严格)"("DisabledEnum"=w231) -> ()  [unwired: 2 in, 2 out]
                    n170 = property on="LAN Port_MPM" class="DigNum (严格)"("DisabledEnum"=w231) -> ()  [unwired: 2 in, 2 out]
                    n171 = property on="LAN Port_MPM 2" class="DigNum (严格)"("DisabledEnum"=w231) -> ()  [unwired: 2 in, 2 out]
                    n172 = property on="IP Address_MPM 2" class="Str"("DisabledEnum"=w231) -> ()  [unwired: 2 in, 2 out]
                    n173 = property on="IP Address_MPM" class="Str"("DisabledEnum"=w231) -> ()  [unwired: 2 in, 2 out]
                  }
                }
              }
            }
          }
          event Panel Close? {
            n174 = event-data() -> ()  [unwired: 1 in, 4 out]
            n175 = event-data("Discard?"=TRUE ("放弃？")) -> ()  [unwired: 1 in, 1 out]
            "Boolean" <- FALSE
          }
        }
      }
    }
  }
  "Address Cluster out" <- w1
  n176 = call <vilib>:"General Error Handler.vi"("error in (no error)"=w4) -> ("error out"=→"错误输出":errorcluster)  [unwired: 10 in, 4 out]
